vi "Read Ultrasonic.vi"() -> (2 "distance":dbl)   [LabVIEW 2011]
panel:
  out "raw distance":dbl
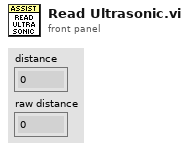
[diagram p1: front panel]
types:
  T1 = typedef "WPI_CounterDevRef.ctl" = cluster{"DevStatus":errorcluster, "CntIndex":T2}
  T2 = typedef "FPGA_CounterCtrSystemIndex.ctl" = enum8{"Ctr 0", "Ctr 1", "Ctr 2", "Ctr 3", "Ctr 4", "Ctr 5", "Ctr 6", "Ctr 7", "Invalid"}
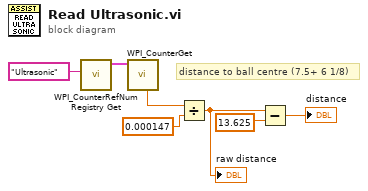
[diagram p0: block diagram]
diagram:
  # "distance to ball centre (7.5+ 6 1/8)"
  n1 = call <vilib>:"WPI_CounterRefNum Registry Get.vi"("refnum name"="Ultrasonic") -> ("CounterDevRef"=w4:T1)  [unwired: 9 in, 1 out]
  n2 = call <vilib>:"WPI_CounterGet.vi"("CounterDevRef in"=w4) -> ("Period (sec)"=w3:dbl)  [unwired: 5 in, 5 out]
  n3 = Divide(x=w3, y=0.000147) -> (x/y=w1:dbl)
  "raw distance" <- w1
  n4 = Subtract(x=w1, y=13.625) -> (x-y=→"distance":dbl)
